vi "ServerRead.vi"(8 "timeout \nms":i32=-1, 11 "port":u16) -> (0 "error out":cluster{"status":bool, i32, "source":string}, 2 "Output Data":string, 3 "connection\n ID out":refnum<k5>)   [LabVIEW 2023]
panel:
  # "Output"
  # "Input"
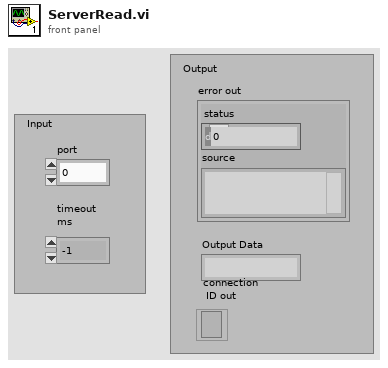
[diagram p1: front panel]
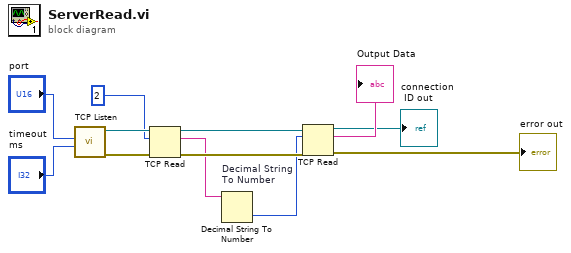
[diagram p0: block diagram]
diagram:
  n1 = call <vilib>:"TCP Listen.vi"("timeout ms (wait forever: -1)"="timeout \nms", "port"="port") -> ("error out"=w10:errorcluster, "connection ID"=w12:refnum<k5>)  [unwired: 5 in, 3 out]
  n2 = TCP Read(connection ID=w12, bytes to read=2, error in (no error)=w10) -> (connection ID out=w11:refnum<k5>, data out=w7:string, error out=w9:errorcluster)  [unwired: 2 in]
  n3 = Decimal String To Number "Decimal String \nTo Number"(string=w7) -> (number=w6:i32)  [unwired: 2 in, 1 out]
  n4 = TCP Read(connection ID=w11, bytes to read=w6, error in (no error)=w9) -> (connection ID out=→"connection\n ID out":refnum<k5>, data out=→"Output Data":string, error out=→"error out":errorcluster)  [unwired: 2 in]
